vi "CSM_pos_0@9.vi"(4 "error in (no error)":errorcluster caption="err in", 5 "q":dbl, 6 "T":dbl, 7 "Pu":dbl) -> (0 "error out":errorcluster caption="err out", 3 "Cpos":dbl)   [LabVIEW 2010, in "lv_07.lvlib"]
doc: "Calcule le coût de possession (Cpos) en fonction de Pu et T --> Cpos =(q/2).Pu.T"
uses:
  lv_07.lvlib
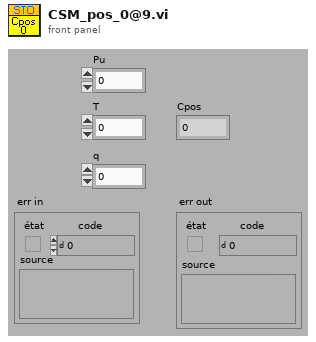
[diagram p1: front panel]
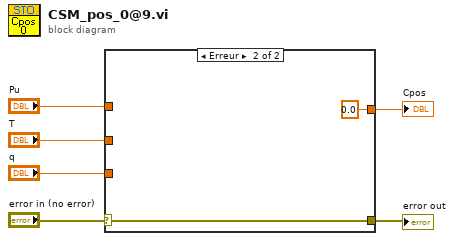
[diagram p0: block diagram]
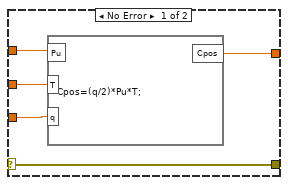
[diagram p2: hidden frame]
diagram:
  n1 = case shown="Erreur" "error in (no error)" {
    selector: "error in (no error)" -> [w7 w13]
    tunnel: [w7 w13] -> w5
    tunnel: [w11 0.0 ("Cpos")] -> w4
    tunnel: "Pu" -> [w10 _]
    tunnel: "T" -> [w9 _]
    tunnel: "q" -> [w8 _]
    frame No Error {
      n2 = formula code="Cpos=(q/2)*Pu*T;"("Pu"=w10, "T"=w9, "q"=w8) -> ("Cpos"=w11:dbl)
    }
    frame Error {
    }
  }
  "Cpos" <- w4
  "error out" <- w5
